vi "read multi-TIFF files(subVI).vi"(3 "file path (use dialog)":path=path "F:/大学/experiment/ViFFI/新しいフォルダー/testss.tif") -> (1 "image data":u16[][][](array[numeric]))   [LabVIEW 2024] (continued)
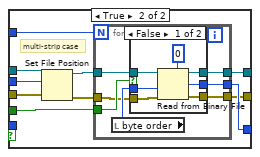
[diagram p2: hidden frame]
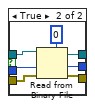
[diagram p3: hidden frame]
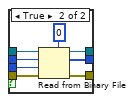
[diagram p4: hidden frame]
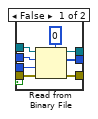
[diagram p5: hidden frame]
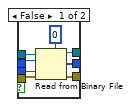
[diagram p6: hidden frame]
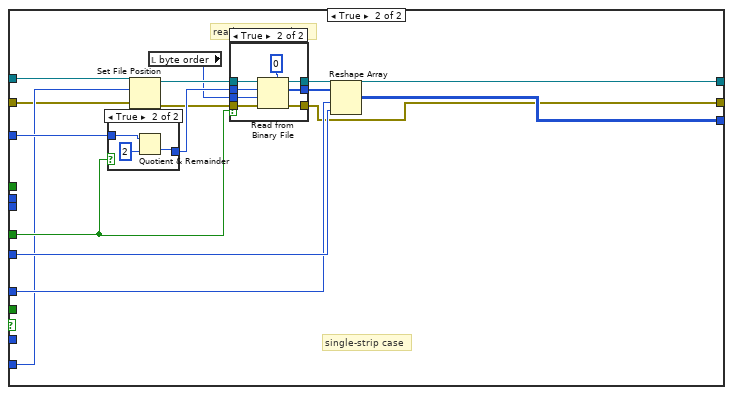
[diagram p7: hidden frame]
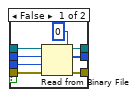
[diagram p8: hidden frame]
      n14 = Search 1D Array(1D array=i32[] [254, 256, 257, 258, 259, 262, 263, 264, 265, 266, 270, 271, 272, 273, 274, 277, 278, 279, 280, 281, 282, 283, 284, 290, 291, 296, 305, 306, 315, 316, 320, 338, 33432] ("Array 2"), element=w67) -> (index of element=w65:i32)  [unwired: 1 in]
      n15 = Index Array(array=string[] ["NewSubfileType", "ImageWidth", "ImageLength", "BitsPerSample", "Compression", "PhotometricInterpretation", "Thresholding", "CellWidth", "CellLength", "FillOrder", "ImageDescription", "Make", "Model", "StripOffsets", "Orientation", "SamplesPerPixel", "RowsPerStrip", "StripByteCounts", "MinSampleValue", "MaxSampleValue", "XResolusion", "YResolusion", "PlanarConfiguration", "GrayResponseUnit", "GrayResponseCurve", "ResolutionUnit", "Software", "DateTime", "Artist", "HostComputer", "ColorMap", "ExtraSamples", "Copyright"] ("Array 3"), index=w65) -> (element=w64:string)
      n16 = Read from Binary File(5:u32 0, 8:w61, 9:w69, 11:w76) -> (0:w60:errorcluster, 2:w71:u32, 3:w75:refnum<file>)  [unwired: 2 in, 1 out]
      n17 = Read from Binary File(5:u32 0, 8:w60, 9:w69, 11:w75) -> (0:w59:errorcluster, 2:w70:u32, 3:w74:refnum<file>)  [unwired: 2 in, 1 out]
    }
    n18 = Build Array(w50, w49, w48, w47) -> (w41:u32[][])
    n19 = Read from Binary File(5:u32 0, 8:w35, 9:w42, 11:w51) -> (0:w34:errorcluster, 2:w52:u32, 3:w54:refnum<file>)  [unwired: 2 in, 1 out]
    n20 = Equal To 0?(x=w52) -> (x = 0?=w53:bool)
    n21 = Transpose 2D Array(2D array=w41) -> (transposed array=w39:u32[][])
    n22 = Set File Position(offset (in bytes) (0)=w52, refnum=w54, error in=w34) -> (refnum out=w44:refnum<file>, error out=w33:errorcluster)  [unwired: 1 in]
    n23 = Bundle(w40, w39) -> (w38:cluster{string[], u32[][]})  [unwired: 1 in]
  }
  "IFD" <- w22
  n24 = Increment(x=w21) -> (x+1=w11:i32)
  "num of frames" <- w11
  n25 = for {
    N: w11 -> [_]
    tunnel: w14 -> [w124]
    tunnel: w13 -> [w92]
    tunnel: [w89] -> w10 mode=indexing
    tunnel: w4 -> [w85]
    tunnel: [w83] -> w3
    tunnel: [w82] -> w2
    i -> [w90]
    # "8bit or 16bit"
    n26 = Index Array(array=w92, index (dim 0)=w90) -> (element=w121:u32[][])  [unwired: 2 in]
    n27 = Index Array(array=w121, index (row)=0) -> (element=w120:u32[])  [unwired: 1 in]
    n28 = Search 1D Array(1D array=w120, element=u32 279) -> (index of element=w99:i32)  [unwired: 1 in]
    n29 = Search 1D Array(1D array=w120, element=u32 258) -> (index of element=w103:i32)  [unwired: 1 in]
    n30 = Search 1D Array(1D array=w120, element=u32 256) -> (index of element=w102:i32)  [unwired: 1 in]
    n31 = Search 1D Array(1D array=w120, element=u32 257) -> (index of element=w101:i32)  [unwired: 1 in]
    n32 = Search 1D Array(1D array=w120, element=u32 273) -> (index of element=w100:i32)  [unwired: 1 in]
    n33 = Search 1D Array(1D array=w120, element=u32 277) -> (index of element=w118:i32)  [unwired: 1 in]
    n34 = Index Array(array=w121, index (col)=w99) -> (element=w106:u32[])  [unwired: 1 in]
    "StripByteCounts" <- w106
    n35 = Index Array(array=w121, index (row)=3 ("disabled index (row)"), index (col)=w103) -> (element=w123:u32)
    "BitsPerSample" <- w123
    n36 = Index Array(array=w121, index (row)=3 ("disabled index (row)"), index (col)=w102) -> (element=w116:u32)
    "ImageWidth" <- w116
    n37 = Index Array(array=w121, index (row)=3 ("disabled index (row)"), index (col)=w101) -> (element=w115:u32)
    "ImageLength" <- w115
    n38 = Index Array(array=w121, index (col)=w100) -> (element=w108:u32[])  [unwired: 1 in]
    "StripOffsets" <- w108
    n39 = Index Array(array=w121, index (row)=3 ("disabled index (row)"), index (col)=w118) -> (element=→"Num of colors":u32)
    n40 = Index Array(array=w108) -> (element #2=w110:u32, element #3=w113:u32, element #4=w87:u32)  [unwired: 4 in, 1 out]
    n41 = Index Array(array=w106) -> (element #2=w112:u32, element #3=w128:u32, element #4=w86:u32)  [unwired: 4 in, 1 out]
    n42 = Equal?(x=w112, y=u32 4) -> (x = y?=w131:bool)
    n43 = Equal?(x=w110, y=u32 4) -> (x = y?=w132:bool)
    n44 = Greater?(x=w128, y=u32 1) -> (0:w130:bool)
    n45 = case shown="False" w130 {
      tunnel: w124 -> [w135 w145]
      tunnel: [w135 w143] -> w125
      tunnel: w128 -> [_ w142]
      tunnel: w86 -> [_ w141]
      tunnel: [w134 w140] -> w126
      tunnel: w86 -> [w134 _]
      tunnel: w131 -> [_ w139]
      tunnel: w85 -> [w133 w138]
      tunnel: [w133 w136] -> w84
      frame False {
        # "single-strip case"
      }
      frame True {
        # "multi-strip case"
        n46 = Set File Position(offset (in bytes) (0)=w141, refnum=w145, error in=w138) -> (refnum out=w144:refnum<file>, error out=w137:errorcluster)  [unwired: 1 in]
        n47 = for {
          N: w142 -> [_]
          tunnel: [w149] -> w140
          tunnel: w144 -> [w152]
          tunnel: [w151] -> w143
          tunnel: w139 -> [w148]
          tunnel: w137 -> [w147]
          tunnel: [w146] -> w136
          n48 = local read "byte order"() -> (w150:T1)
          n49 = case shown="False" w148 {
            tunnel: w152 -> [w159 w166]
            tunnel: [w157 w165] -> w151
            tunnel: w150 -> [w158 w164]
            tunnel: [w156 w163] -> w149
            tunnel: w147 -> [w154 w161]
            tunnel: [w153 w160] -> w146
            frame False {
              n50 = Read from Binary File(5:u16 0, 8:w154, 9:w158, 11:w159) -> (0:w153:errorcluster, 2:w156:u16, 3:w157:refnum<file>)  [unwired: 2 in, 1 out]
            }
            frame True {
              n51 = Read from Binary File(5:u32 0, 8:w161, 9:w164, 11:w166) -> (0:w160:errorcluster, 2:w163:u32, 3:w165:refnum<file>)  [unwired: 2 in, 1 out]
            }
          }
        }
      }
    }
    n52 = Equal?(x=u32 1, y=w113) -> (x = y?=w88:bool)
    n53 = Equal?(x=16, y=w123) -> (x = y?=w127:bool)
    n54 = case shown="False" w88 {
      tunnel: w125 -> [w193 w258]
      tunnel: [w190 w260] -> w89
      tunnel: w86 -> [w187 _]
      tunnel: w113 -> [w186 _]
      tunnel: w87 -> [w185 w257]
      tunnel: w128 -> [w184 _]
      tunnel: w131 -> [w182 _]
      tunnel: w127 -> [w178 w259]
      tunnel: w115 -> [_ w264]
      tunnel: w116 -> [_ w265]
      tunnel: w126 -> [_ w262]
      tunnel: w132 -> [w181 _]
      tunnel: [w173 w256] -> w83
      tunnel: w84 -> [w172 w255]
      tunnel: [w167 w253] -> w82
      frame False {
        # "length of each strip"
        # "positions of each strip"
        # "multiple-strip case"
        n55 = local read "byte order"() -> (w183:T1)
        n56 = Set File Position(offset (in bytes) (0)=w185, refnum=w193, error in=w172) -> (refnum out=w192:refnum<file>, error out=w171:errorcluster)  [unwired: 1 in]
        n57 = case shown="False" w181 {
          tunnel: w192 -> [w201 w209]
          tunnel: [w199 w208] -> w191
          tunnel: [w200 w207] -> w188
          tunnel: w186 -> [w198 w206]
          tunnel: w183 -> [w197 w205]
          tunnel: w171 -> [w195 w203]
          tunnel: [w194 w202] -> w170
          frame False {
            n58 = Read from Binary File(5:u16 0, 8:w195, 9:w197, 10:w198, 11:w201) -> (0:w194:errorcluster, 2:w199:u16[], 3:w200:refnum<file>)  [unwired: 1 in, 1 out]
          }
          frame True {
            n59 = Read from Binary File(5:u32 0, 8:w203, 9:w205, 10:w206, 11:w209) -> (0:w202:errorcluster, 2:w208:u32[], 3:w207:refnum<file>)  [unwired: 1 in, 1 out]
          }
        }
        n60 = Set File Position(offset (in bytes) (0)=w187, refnum=w188, error in=w170) -> (refnum out=w189:refnum<file>, error out=w169:errorcluster)  [unwired: 1 in]
        n61 = case shown="True" w182 {
          tunnel: w189 -> [w217 w225]
          tunnel: [w216 w224] -> w174
          tunnel: w184 -> [w214 w223]
          tunnel: [w215 w222] -> w180
          tunnel: w183 -> [w213 w221]
          tunnel: w169 -> [w211 w219]
          tunnel: [w210 w218] -> w168
          frame False {
            n62 = Read from Binary File(5:u16 0, 8:w211, 9:w213, 10:w214, 11:w217) -> (0:w210:errorcluster, 2:w215:u16[], 3:w216:refnum<file>)  [unwired: 1 in, 1 out]
          }
          frame True {
            n63 = Read from Binary File(5:u32 0, 8:w219, 9:w221, 10:w223, 11:w225) -> (0:w218:errorcluster, 2:w222:u32[], 3:w224:refnum<file>)  [unwired: 1 in, 1 out]
          }
        }
        n64 = To Long Integer(number=w180) -> (32bit integer=w177:i32[])
        n65 = Quotient & Remainder(x=w177, y=2) -> (floor(x/y)=w175:i32[])  [unwired: 1 out]
        n66 = Select(t=w175, s=w178, f=w177) -> (s? t:f=w176:i32[])
        n67 = for {
          tunnel: w191 -> [w229] mode=indexing
          tunnel: w174 -> [w236]
          tunnel: [w234] -> w173
          tunnel: [w233] -> w190 mode=indexing
          tunnel: w176 -> [w231] mode=indexing
          tunnel: w183 -> [w232]
          tunnel: w178 -> [w230]
          tunnel: w168 -> [w228]
          tunnel: [w226] -> w167
          # "readout strips"
          n68 = Set File Position(offset (in bytes) (0)=w229, refnum=w236, error in=w228) -> (refnum out=w235:refnum<file>, error out=w227:errorcluster)  [unwired: 1 in]
          n69 = case shown="True" w230 {
            tunnel: w235 -> [w243 w252]
            tunnel: [w242 w251] -> w234
            tunnel: [w241 w250] -> w233
            tunnel: w232 -> [w239 w249]
            tunnel: w231 -> [w240 w248]
            tunnel: w227 -> [w238 w245]
            tunnel: [w237 w246] -> w226
            frame False {
              n70 = Read from Binary File(5:u8 0, 8:w238, 9:w239, 10:w240, 11:w243) -> (0:w237:errorcluster, 2:w241:u8[], 3:w242:refnum<file>)  [unwired: 1 in, 1 out]
            }
            frame True {
              n71 = Read from Binary File(5:u16 0, 8:w245, 9:w249, 10:w248, 11:w252) -> (0:w246:errorcluster, 2:w250:u16[], 3:w251:refnum<file>)  [unwired: 1 in, 1 out]
            }
          }
        }
      }
      frame True {
        # "readout image data"
        # "single-strip case"
        n72 = case shown="True" w259 {
          tunnel: w262 -> [w284 w286]
          tunnel: [w284 w285] -> w266
          frame False {
          }
          frame True {
            n73 = Quotient & Remainder(x=w286, y=u16 2) -> (floor(x/y)=w285:u32)  [unwired: 1 out]
          }
        }
        n74 = Set File Position(offset (in bytes) (0)=w257, refnum=w258, error in=w255) -> (refnum out=w267:refnum<file>, error out=w254:errorcluster)  [unwired: 1 in]
        n75 = local read "byte order"() -> (w263:T1)
        n76 = case shown="True" w259 {
          tunnel: w267 -> [w271 w283]
          tunnel: w266 -> [w272 w282]
          tunnel: [w270 w281] -> w256
          tunnel: w263 -> [w273 w280]
          tunnel: [w275 w279] -> w261
          tunnel: w254 -> [w269 w277]
          tunnel: [w268 w276] -> w253
          frame False {
            n77 = Read from Binary File(5:u8 0, 8:w269, 9:w273, 10:w272, 11:w271) -> (0:w268:errorcluster, 2:w275:u8[], 3:w270:refnum<file>)  [unwired: 1 in, 1 out]
          }
          frame True {
            n78 = Read from Binary File(5:u16 0, 8:w277, 9:w280, 10:w282, 11:w283) -> (0:w276:errorcluster, 2:w279:u16[], 3:w281:refnum<file>)  [unwired: 1 in, 1 out]
          }
        }
        n79 = Reshape Array(w261, w264, w265) -> (w260:u16[][])
      }
    }
    "Numeric 2" <- w90
  }
  "image data" <- w10
  n80 = Close File(refnum=w3, error in=w2) -> (error out=→"error out":errorcluster)  [unwired: 1 out]
